vi "Receive Results Object.vi"(8 "error in (no error)":errorcluster, 10 "Results.lvclass":refnum<class "Results.lvclass">, 11 "Server Controller in":refnum<class "Server Controller.lvclass">) -> (0 "error out":errorcluster, 3 "Server Controller out":refnum<class "Server Controller.lvclass">)   [LabVIEW 2016, in "Server Controller.lvlib" / "Server Controller.lvclass"]
uses:
  Server Controller.lvclass
  \\Mac\Home/Documents/MAL-Framework/user.lib/Common Components/Controller/Controller.lvclass
  MAL-Framework/user.lib/Common Components/Results/Results.lvclass
  MAL-Framework/user.lib/Common Components/Controller/Controller.lvclass
  MAL-Framework/user.lib/Common Components/User Interface/Messages/Display Results/Display Results.lvclass
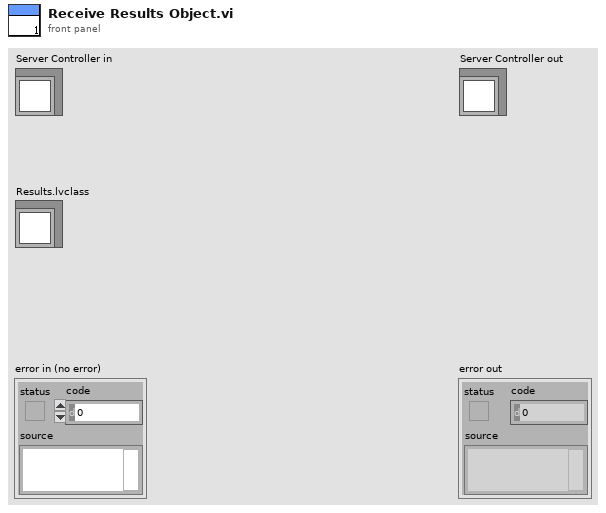
[diagram p1: front panel]
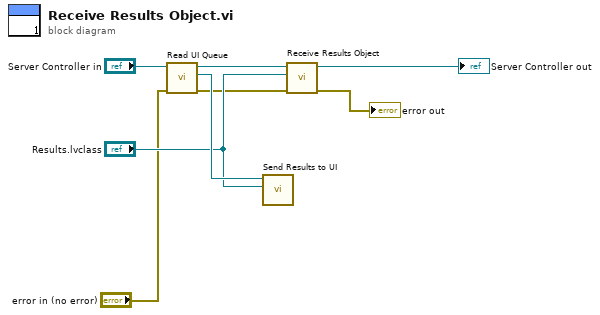
[diagram p0: block diagram]
diagram:
  n1 = call "Read UI Queue.vi"("error in (no error)"="error in (no error)", "UI Controller in"="Server Controller in") -> ("error out"=w1:errorcluster, "UI Queue"=w6:refnum<class "Message Enqueuer.lvclass">, "UI Controller out"=w2:refnum<class "Server Controller.lvclass">)  [unwired: 7 in]
  n2 = call "Send Results to UI.vi"("Results.lvclass"="Results.lvclass", "UI Queue"=w6) -> ()  [unwired: 8 in, 2 out]
  n3 = call-parent "Receive Results Object.vi"("error in (no error)"=w1, "Results.lvclass"="Results.lvclass", "Controller in"=w2) -> ("error out"=→"error out":errorcluster, "Controller out"=→"Server Controller out":refnum<class "Server Controller.lvclass">)  [unwired: 7 in]
